vi "海流计数据上传.vi"(8 "错误输入（无错误）":errorcluster) -> (0 "error out":errorcluster)   [LabVIEW 2016, in "数据传输系统-04.lvlib"]
uses:
  <vilib>/Utility/config.llb/Read Key (String).vi
  <vilib>/Utility/config.llb/Write Key (String).vi
  <vilib>/Utility/config.llb/NI_LVConfig.lvlib
  <vilib>/ptbypt/NI_PtbyPt.lvlib
panel:
  out "读取的时间值":string caption="值"
  out "超时":bool
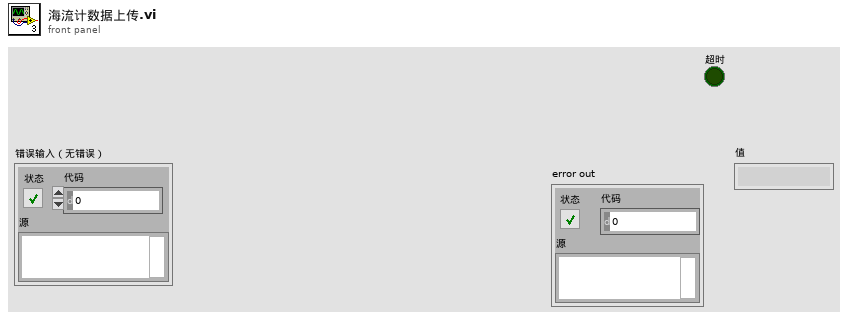
[diagram p1: front panel]
types:
  T1 = enum16{"open", "replace", "create", "open or create", "replace or create", "replace or create with confirmation"}
  T2 = cluster{"setini":string, "sysini":string, "hechaini":string, "actualwrite":string, "actualread":string, "datasent":string, "反控命令信息队列":string, "反控与仪器交互":string}
  T3 = typedef "NI_LVConfig.lvlib/Config Data RefNum.ctl" = refnum<k1>
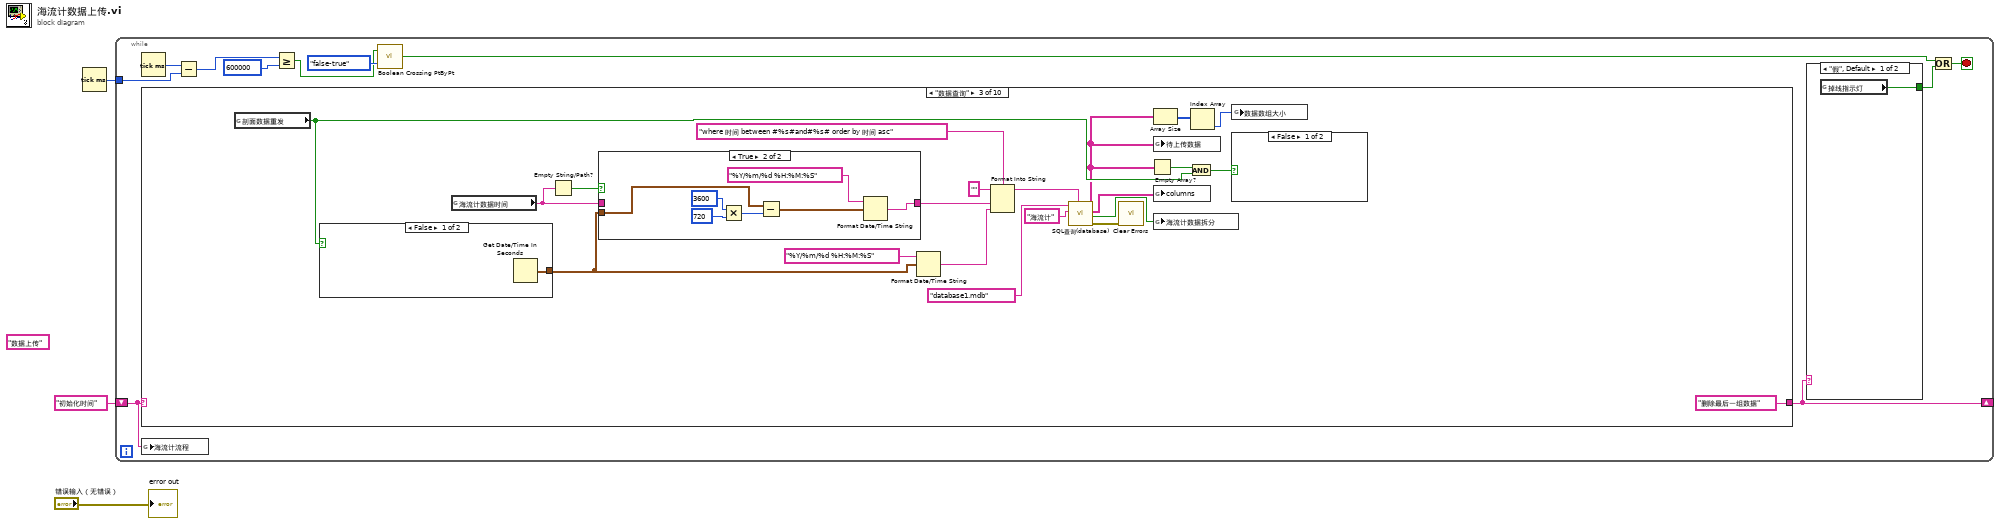
[diagram p0: block diagram]
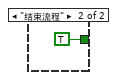
[diagram p2: hidden frame]
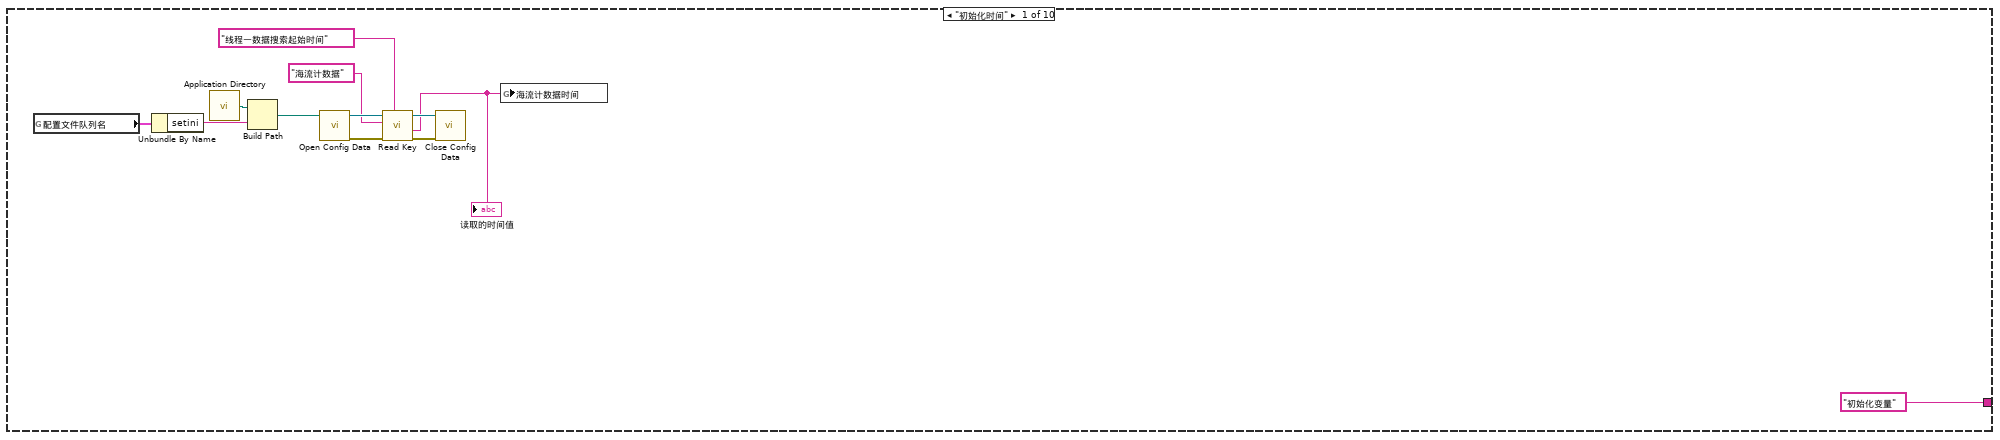
[diagram p3: hidden frame]
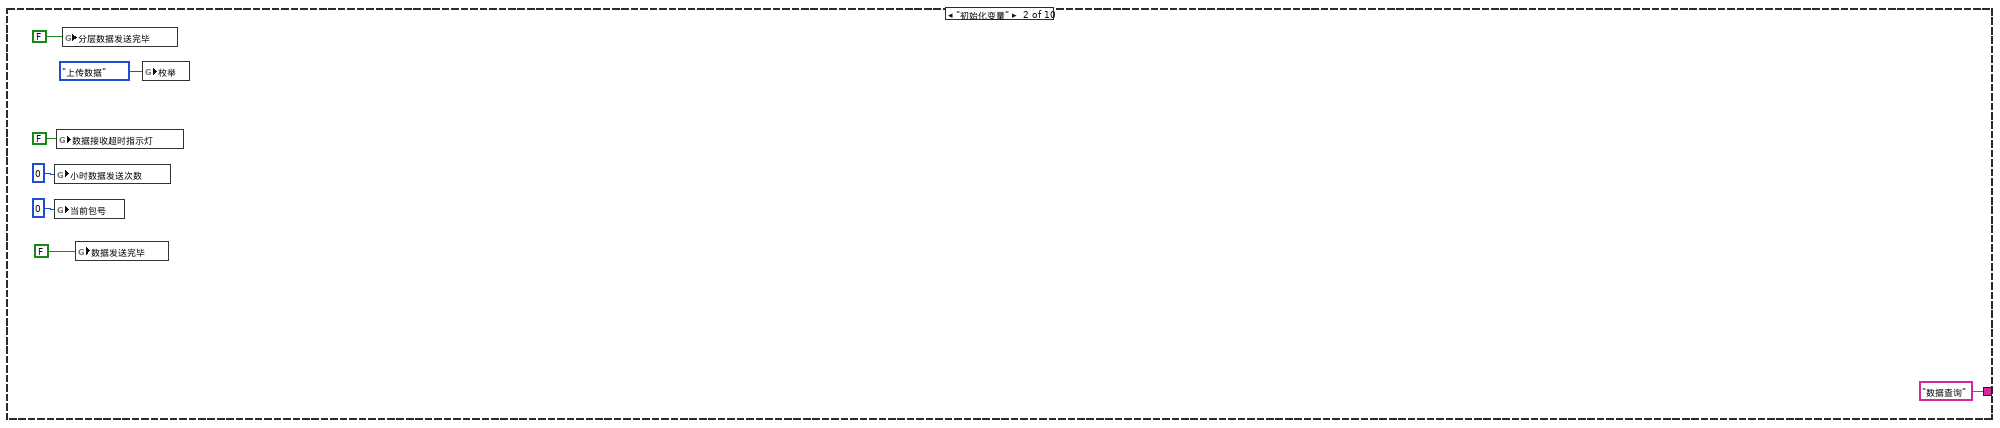
[diagram p4: hidden frame]
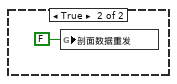
[diagram p5: hidden frame]
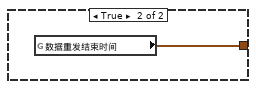
[diagram p7: hidden frame]
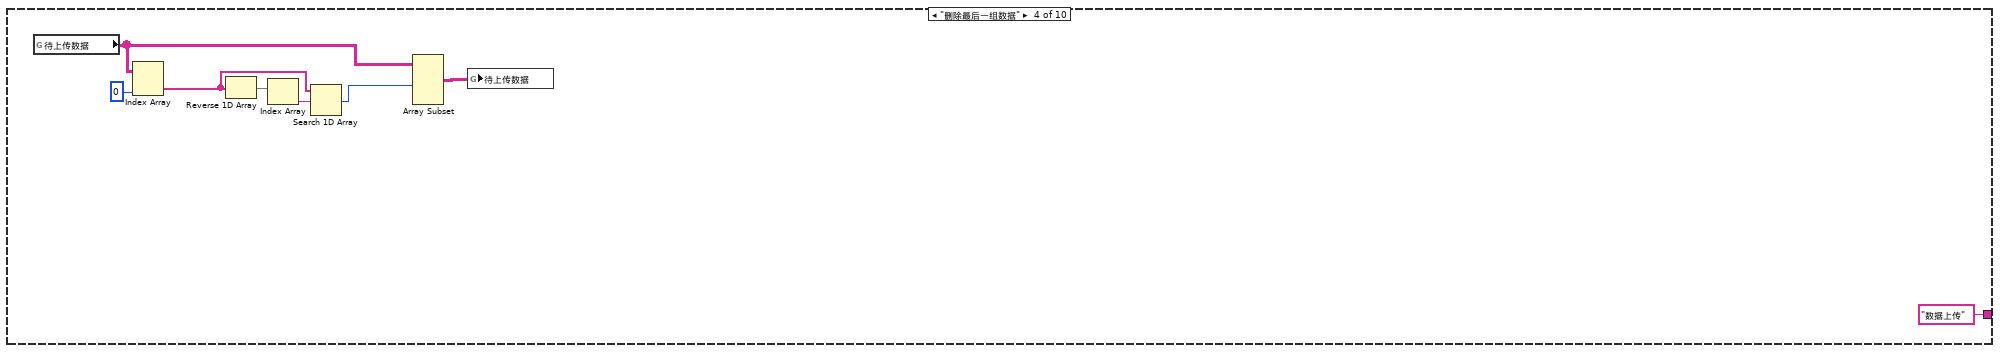
[diagram p8: hidden frame]
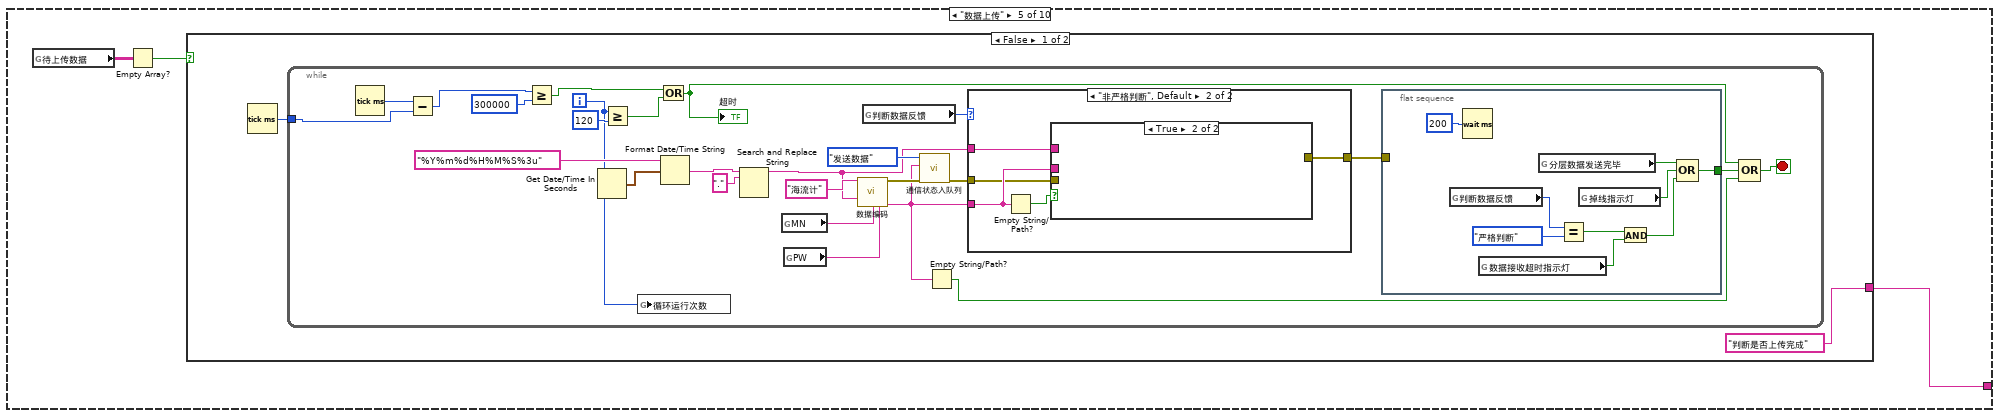
[diagram p9: hidden frame]
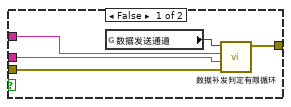
[diagram p11: hidden frame]
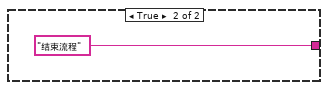
[diagram p12: hidden frame]
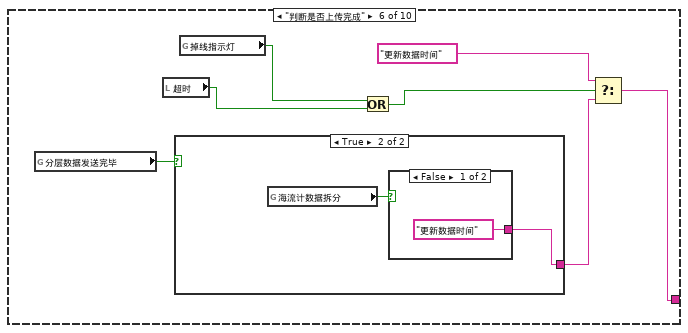
[diagram p13: hidden frame]
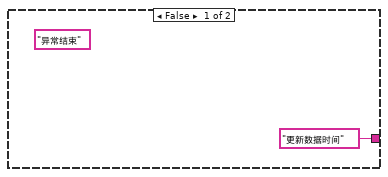
[diagram p14: hidden frame]
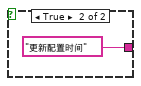
[diagram p15: hidden frame]
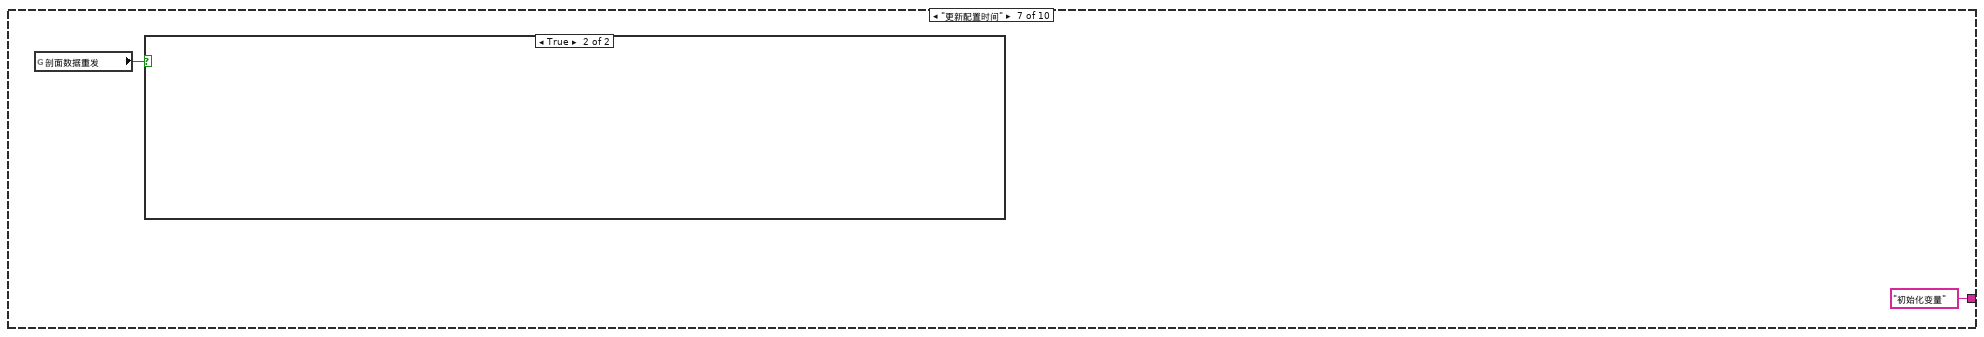
[diagram p16: hidden frame]
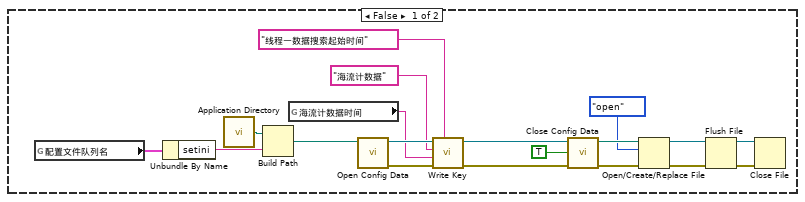
[diagram p17: hidden frame]
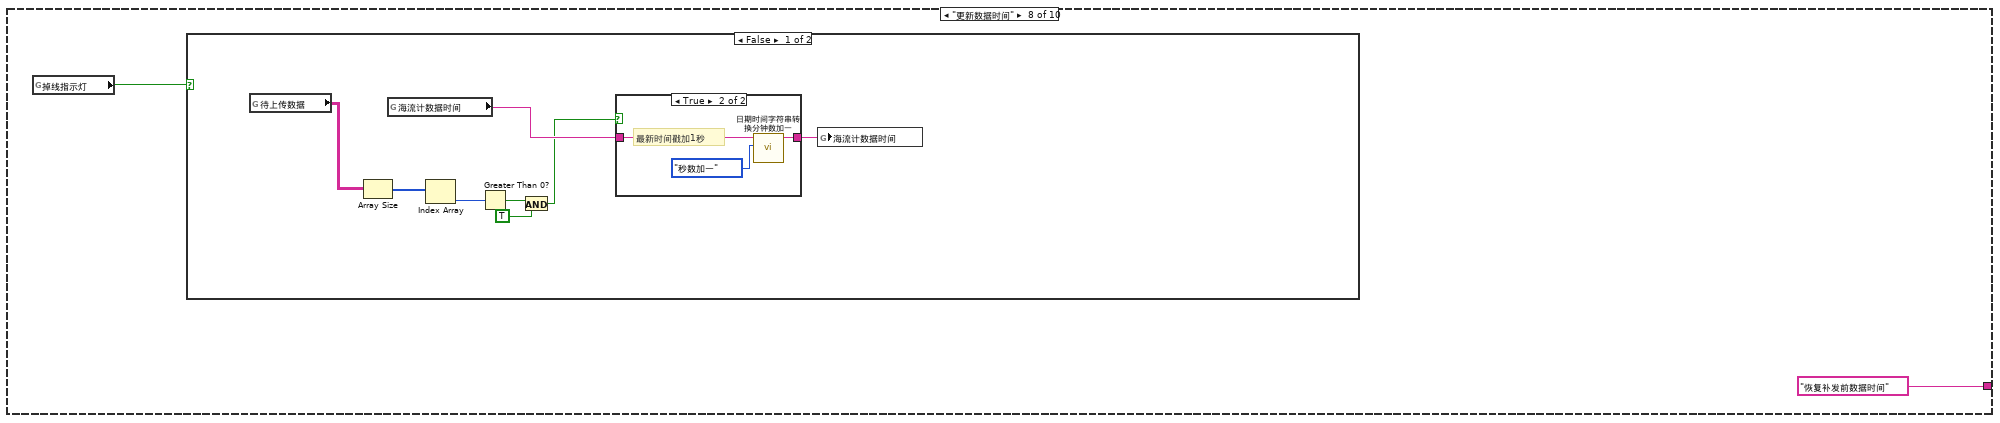
[diagram p18: hidden frame]
diagram:
  (unwired) "数据上传"
  n1 = Tick Count (ms)() -> (millisecond timer value=w2:u32)
  n2 = while {
    shift-right: [w14] -> _
    shift-left: "初始化时间" -> [w13]
    tunnel: w2 -> [w11]
    stop <- w7 stop-if-true
    n3 = Tick Count (ms)() -> (millisecond timer value=w12:u32)
    n4 = case shown="\"数据查询\"" w13 {
      tunnel: ["初始化变量" "数据查询" "删除最后一组数据" "数据上传" w76 w130 "初始化变量" "恢复补发前数据时间" "结束流程" "结束流程"] -> w14
      frame "初始化时间" {
        n5 = global read "全局1.vi" "配置文件队列名"() -> (w28:T2)
        n6 = Unbundle By Name(w28) -> ("setini"=w21:string)
        n7 = call <vilib>:"Application Directory.vi"() -> ("Application Directory"=w22:path)
        n8 = Build Path(base path=w22, name or relative path=w21) -> (appended path=w20:path)
        n9 = call <vilib>:"Open Config Data.vi"("configuration file path"=w20) -> ("error out"=w25:errorcluster, "refnum"=w26:T3)  [unwired: 8 in, 1 out]
        n10 = call-poly <vilib>:"Read Key.vi"("section"="线程一数据搜索起始时间", "error in (no error)"=w25, "key"="海流计数据", "refnum"=w26) -> ("error out"=w23:errorcluster, "value"=w18:string, "refnum out"=w24:T3)  [unwired: 4 in, 1 out]
        "读取的时间值" <- w18
        n11 = call <vilib>:"Close Config Data.vi"("error in (no error)"=w23, "refnum"=w24) -> ()  [unwired: 8 in, 2 out]
        n12 = global write "全局 水样时间.vi" "海流计数据时间"(w18) -> ()
      }
      frame "初始化变量" {
        n13 = global write "全局 小时数据发送次数.vi" "小时数据发送次数"(0 ("小时数据发送次数")) -> ()
        n14 = global write "全局 数据数组大小.vi" "当前包号"(0 ("当前包号")) -> ()
        n15 = global write "全局 数据发送重叠.vi" "数据接收超时指示灯"(FALSE ("数据接收超时指示灯")) -> ()
        n16 = global write "全局 数据数组大小.vi" "分层数据发送完毕"(FALSE ("海流计数据发送完毕")) -> ()
        n17 = global write "全局 数据数组大小.vi" "数据发送完毕"(FALSE ("海流计数据发送完毕")) -> ()
        n18 = global write "全局1.vi" "枚举"(enum16{"返回请求应答", "上传数据", "返回执行结果"}."上传数据" ("枚举")) -> ()
      }
      frame "数据查询" {
        n19 = global read "断电保存全局.vi" "剖面数据重发"() -> (w55:bool)
        n20 = case shown="False" w55 {
          tunnel: [w66 w67] -> w48
          frame False {
            n21 = Get Date/Time In Seconds() -> (seconds since 1Jan1904=w66:timestamp)
          }
          frame True {
            n22 = global read "断电保存全局.vi" "数据重发结束时间"() -> (w67:timestamp)
          }
        }
        n23 = global read "全局 水样时间.vi" "海流计数据时间"() -> (w49:string)
        n24 = Empty String/Path?(string/path=w49) -> (empty?=w47:bool)
        n25 = case shown="True" w47 {
          tunnel: w48 -> [_ w63]
          tunnel: [w58 w59] -> w50
          tunnel: w49 -> [w58 _]
          frame False {
          }
          frame True {
            n26 = Multiply(x=3600, y=720) -> (x*y=w62:i32)
            n27 = Subtract(x=w63, y=w62) -> (x-y=w60:timestamp)
            n28 = Format Date/Time String(time format string (%c)="%Y/%m/%d %H:%M:%S" ("时间格式字符串(%c)"), seconds (now)=w60) -> (date/time string=w59:string)  [unwired: 1 in]
          }
        }
        n29 = Format Date/Time String(time format string (%c)="%Y/%m/%d %H:%M:%S" ("时间格式字符串(%c)"), seconds (now)=w48) -> (date/time string=w41:string)  [unwired: 1 in]
        n30 = Format Into String(format string="where 时间 between #%s#and#%s# order by 时间 asc" ("condition"), initial string="" ("初始字符串"), w50, w41) -> (resulting string=w42:string)  [unwired: 1 in, 1 out]
        n31 = call "SQL查询(database).vi"("condition"=w42, "table输入"="海流计", "database"="database1.mdb") -> ("error out"=w45:errorcluster, "拆分数据"=w52:bool, "columns输出"=w51:string[], "data"=w53:string[][])  [unwired: 5 in]
        n32 = call <vilib>:"Clear Errors.vi"("error in (no error)"=w45) -> ()  [unwired: 5 in, 2 out]
        n33 = Empty Array?(array=w53) -> (empty?=w54:bool)
        n34 = Array Size(array=w53) -> (size(s)=w43:i32[])
        n35 = global write "全局 所有参数.vi" "待上传数据"(w53) -> ()
        n36 = global write "全局 所有参数.vi" "columns"(w51) -> ()
        n37 = global write "全局 所有参数.vi" "海流计数据拆分"(w52) -> ()
        n38 = And(x=w54, y=w55) -> (x .and. y?=w56:bool)
        n39 = Index Array(array=w43) -> (element=w44:i32)  [unwired: 1 in]
        n40 = global write "全局 数据数组大小.vi" "数据数组大小"(w44) -> ()
        n41 = case shown="False" w56 {
          frame False {
          }
          frame True {
            n42 = global write "断电保存全局.vi" "剖面数据重发"(FALSE ("剖面数据重发")) -> ()
          }
        }
      }
      frame "删除最后一组数据" {
        n43 = global read "全局 所有参数.vi" "待上传数据"() -> (w71:string[][])
        n44 = Index Array(array=w71, index (col)=0 ("禁用的索引 (列)")) -> (element=w72:string[])  [unwired: 1 in]
        n45 = Reverse 1D Array(array=w72) -> (reversed array=w74:string[])
        n46 = Index Array(array=w74) -> (element=w73:string)  [unwired: 1 in]
        n47 = Search 1D Array(1D array=w72, element=w73) -> (index of element=w68:i32)  [unwired: 1 in]
        n48 = Array Subset(array=w71, length (row)=w68) -> (w70:string[][])  [unwired: 3 in]
        n49 = global write "全局 所有参数.vi" "待上传数据"(w70) -> ()
      }
      frame "数据上传" {
        n50 = global read "全局 所有参数.vi" "待上传数据"() -> (w77:string[][])
        n51 = Empty Array?(array=w77) -> (empty?=w78:bool)
        n52 = case shown="False" w78 {
          tunnel: ["判断是否上传完成" "结束流程"] -> w76
          frame False {
            n53 = Tick Count (ms)() -> (millisecond timer value=w80:u32)
            n54 = while {
              tunnel: w80 -> [w90]
              i -> [w81]
              stop <- w84 stop-if-true
              n55 = Tick Count (ms)() -> (millisecond timer value=w91:u32)
              n56 = Subtract(x=w91, y=w90) -> (x-y=w92:u32)
              n57 = Greater Or Equal?(x=w92, y=u32 300000) -> (x >= y?=w87:bool)
              n58 = Get Date/Time In Seconds() -> (seconds since 1Jan1904=w104:timestamp)
              n59 = Greater Or Equal?(x=w81, y=120) -> (x >= y?=w86:bool)
              n60 = global write "全局 水样时间.vi" "循环运行次数"(w81) -> ()
              n61 = Or(x=w87, y=w86) -> (x .or. y?=w85:bool)
              "超时" <- w85
              n62 = Format Date/Time String(time format string (%c)="%Y%m%d%H%M%S%3u" ("时间格式字符串(%c)"), seconds (now)=w104) -> (date/time string=w103:string)  [unwired: 1 in]
              n63 = Search and Replace String(input string=w103, search string="." ("搜索字符串")) -> (result string=w96:string)  [unwired: 6 in, 3 out]
              n64 = global read "断电保存全局.vi" "MN"() -> (w98:string)
              n65 = global read "断电保存全局.vi" "PW"() -> (w101:string)
              n66 = call "数据编码.vi"("table输入"="海流计" ("新元素/子数组"), "QN"=w96, "MN"=w98, "PW"=w101) -> ("错误常量"=w100:errorcluster, "通讯包字符串"=w83:string)  [unwired: 10 in]
              n67 = global read "断电保存全局.vi" "判断数据反馈"() -> (w95:enum16{"非严格判断", "严格判断", "不判断"})
              n68 = call "通信状态入队列.vi"("错误输入（无错误）"=w100, "发送报文"=w83, "枚举"=enum16{"打开连接", "发送数据", "读取数据", "数据处理", "关闭连接"}."发送数据") -> ("错误输出"=w97:errorcluster)  [unwired: 8 in]
              n69 = Empty String/Path?(string/path=w83) -> (empty?=w82:bool)
              n70 = case shown="\"非严格判断\", Default" w95 {
                tunnel: [_ w120] -> w94
                tunnel: w83 -> [_ w119]
                tunnel: w96 -> [_ w118]
                tunnel: w97 -> [_ w116]
                frame "不判断" {
                }
                frame "非严格判断", Default {
                  n71 = Empty String/Path?(string/path=w119) -> (empty?=w117:bool)
                  n72 = case shown="True" w117 {
                    tunnel: [w125 _] -> w120
                    tunnel: w119 -> [w124 _]
                    tunnel: w118 -> [w122 _]
                    tunnel: w116 -> [w121 _]
                    frame False {
                      n73 = global read "断电保存全局.vi" "数据发送通道"() -> (w123:enum16{"TCP", "VISA"})
                      n74 = call "数据补发判定有限循环.vi"("错误输入（无错误）"=w121, "数据输入"=w124, "QN"=w122, "数据发送通道"=w123) -> ("error out"=w125:errorcluster)  [unwired: 7 in]
                    }
                    frame True {
                    }
                  }
                }
              }
              n75 = flat-sequence {
                tunnel: w94 -> [_]
                tunnel: [w110] -> w89
                frame #0 {
                  n76 = global read "断电保存全局.vi" "判断数据反馈"() -> (w114:enum16{"非严格判断", "严格判断", "不判断"})
                  n77 = Wait (ms)(milliseconds to wait=u32 200 ("等待时间（毫秒）")) -> ()  [unwired: 1 out]
                  n78 = global read "全局 数据发送重叠.vi" "数据接收超时指示灯"() -> (w107:bool)
                  n79 = global read "全局 数据数组大小.vi" "分层数据发送完毕"() -> (w109:bool)
                  n80 = Equal?(x=w114, y=enum16{"非严格判断", "严格判断", "不判断"}."严格判断") -> (x = y?=w112:bool)
                  n81 = global read "全局 数据发送重叠.vi" "掉线指示灯"() -> (w108:bool)
                  n82 = And(x=w112, y=w107) -> (x .and. y?=w111:bool)
                  n83 = Compound Arithmetic op=OR ("复合运算")(w109, w108, w111) -> (w110:bool)
                }
              }
              n84 = Compound Arithmetic op=OR ("复合运算")(w85, w89, w82) -> (w84:bool)
            }
          }
          frame True {
          }
        }
      }
      frame "判断是否上传完成" {
        n85 = global read "全局 数据数组大小.vi" "分层数据发送完毕"() -> (w133:bool)
        n86 = local read "超时"() -> (w128:bool)
        n87 = case shown="True" w133 {
          tunnel: ["更新数据时间" w135] -> w131
          frame False {
            (unwired) "异常结束"
          }
          frame True {
            n88 = global read "全局 所有参数.vi" "海流计数据拆分"() -> (w136:bool)
            n89 = case shown="False" w136 {
              tunnel: ["更新数据时间" "更新配置时间"] -> w135
              frame False {
              }
              frame True {
              }
            }
          }
        }
        n90 = global read "全局 数据发送重叠.vi" "掉线指示灯"() -> (w129:bool)
        n91 = Or(x=w129, y=w128) -> (x .or. y?=w127:bool)
        n92 = Select(t="更新数据时间", s=w127, f=w131) -> (s? t:f=w130:string)
      }
      frame "更新配置时间" {
        n93 = global read "断电保存全局.vi" "剖面数据重发"() -> (w140:bool)
        n94 = case shown="True" w140 {
          frame False {
            n95 = global read "全局1.vi" "配置文件队列名"() -> (w143:T2)
            n96 = Unbundle By Name(w143) -> ("setini"=w144:string)
            n97 = call <vilib>:"Application Directory.vi"() -> ("Application Directory"=w153:path)
            n98 = Build Path(base path=w153, name or relative path=w144) -> (appended path=w154:path)
            n99 = global read "全局 水样时间.vi" "海流计数据时间"() -> (w145:string)
            n100 = call <vilib>:"Open Config Data.vi"("configuration file path"=w154) -> ("error out"=w156:errorcluster, "refnum"=w155:T3)  [unwired: 8 in, 1 out]
            n101 = call-poly <vilib>:"Write Key.vi"("section"="线程一数据搜索起始时间", "error in (no error)"=w156, "value"=w145, "key"="海流计数据", "refnum"=w155) -> ("error out"=w158:errorcluster, "refnum out"=w157:T3)  [unwired: 4 in, 1 out]
            n102 = call <vilib>:"Close Config Data.vi"("error in (no error)"=w158, "write file if changed (T)"=TRUE, "refnum"=w157) -> ("error out"=w146:errorcluster, "file path"=w147:path)  [unwired: 7 in]
            n103 = Open/Create/Replace File(file path (use dialog)=w147, error in=w146, operation (0:open)=T1."open" ("操作(0:open)")) -> (refnum out=w149:refnum<file>, error out=w148:errorcluster)  [unwired: 3 in, 1 out]
            n104 = Flush File(refnum=w149, error in=w148) -> (refnum out=w150:refnum<file>, error out=w151:errorcluster)
            n105 = Close File(refnum=w150, error in=w151) -> ()  [unwired: 2 out]
          }
          frame True {
          }
        }
      }
      frame "更新数据时间" {
        n106 = global read "全局 数据发送重叠.vi" "掉线指示灯"() -> (w160:bool)
        n107 = case shown="False" w160 {
          frame False {
            n108 = global read "全局 所有参数.vi" "待上传数据"() -> (w163:string[][])
            n109 = Array Size(array=w163) -> (size(s)=w166:i32[])
            n110 = global read "全局 水样时间.vi" "海流计数据时间"() -> (w169:string)
            n111 = Index Array(array=w166) -> (element=w167:i32)  [unwired: 1 in]
            n112 = Greater Than 0?(x=w167) -> (x > 0?=w165:bool)
            n113 = And(x=w165, y=TRUE) -> (x .and. y?=w162:bool)
            n114 = case shown="True" w162 {
              tunnel: [w170 w173] -> w168
              tunnel: w169 -> [w170 w172]
              frame False {
              }
              frame True {
                # "最新时间戳加1秒"
                n115 = call "日期时间字符串转换分钟数加一.vi"("枚举"=enum16{"分钟数加一", "秒数加一", "小时数加一"}."秒数加一", "data[0]"=w172) -> ("日期/时间字符串"=w173:string)  [unwired: 9 in]
              }
            }
            n116 = global write "全局 水样时间.vi" "海流计数据时间"(w168) -> ()
          }
          frame True {
          }
        }
      }
      frame "恢复补发前数据时间" {
        n117 = global read "断电保存全局.vi" "剖面数据重发"() -> (w175:bool)
        n118 = case shown="False" w175 {
          frame False {
            n119 = global read "全局1.vi" "配置文件队列名"() -> (w178:T2)
            n120 = Unbundle By Name(w178) -> ("setini"=w179:string)
            n121 = call <vilib>:"Application Directory.vi"() -> ("Application Directory"=w188:path)
            n122 = Build Path(base path=w188, name or relative path=w179) -> (appended path=w189:path)
            n123 = global read "全局 水样时间.vi" "海流计数据时间"() -> (w180:string)
            n124 = call <vilib>:"Open Config Data.vi"("configuration file path"=w189) -> ("error out"=w191:errorcluster, "refnum"=w190:T3)  [unwired: 8 in, 1 out]
            n125 = call-poly <vilib>:"Write Key.vi"("section"="线程一数据搜索起始时间", "error in (no error)"=w191, "value"=w180, "key"="海流计数据", "refnum"=w190) -> ("error out"=w193:errorcluster, "refnum out"=w192:T3)  [unwired: 4 in, 1 out]
            n126 = call <vilib>:"Close Config Data.vi"("error in (no error)"=w193, "write file if changed (T)"=TRUE, "refnum"=w192) -> ("error out"=w181:errorcluster, "file path"=w182:path)  [unwired: 7 in]
            n127 = Open/Create/Replace File(file path (use dialog)=w182, error in=w181, operation (0:open)=T1."open" ("操作(0:open)")) -> (refnum out=w184:refnum<file>, error out=w183:errorcluster)  [unwired: 3 in, 1 out]
            n128 = Flush File(refnum=w184, error in=w183) -> (refnum out=w185:refnum<file>, error out=w186:errorcluster)
            n129 = Close File(refnum=w185, error in=w186) -> ()  [unwired: 2 out]
          }
          frame True {
            n130 = global write "断电保存全局.vi" "剖面数据重发"(FALSE ("剖面数据重发")) -> ()
            n131 = global read "全局1.vi" "配置文件队列名"() -> (w195:T2)
            n132 = Unbundle By Name(w195) -> ("setini"=w203:string)
            n133 = call <vilib>:"Application Directory.vi"() -> ("Application Directory"=w202:path)
            n134 = Build Path(base path=w202, name or relative path=w203) -> (appended path=w204:path)
            n135 = call <vilib>:"Open Config Data.vi"("configuration file path"=w204) -> ("error out"=w199:errorcluster, "refnum"=w198:T3)  [unwired: 8 in, 1 out]
            n136 = call-poly <vilib>:"Read Key.vi"("section"="线程一数据搜索起始时间", "error in (no error)"=w199, "key"="海流计数据", "refnum"=w198) -> ("error out"=w201:errorcluster, "value"=w206:string, "refnum out"=w200:T3)  [unwired: 4 in, 1 out]
            n137 = call <vilib>:"Close Config Data.vi"("error in (no error)"=w201, "refnum"=w200) -> ()  [unwired: 8 in, 2 out]
            n138 = global write "全局 水样时间.vi" "海流计数据时间"(w206) -> ()
          }
        }
      }
      frame "结束流程", Default {
      }
    }
    n139 = global write "全局 水样时间.vi" "海流计流程"(w13) -> ()
    n140 = Subtract(x=w12, y=w11) -> (x-y=w10:u32)
    n141 = Greater Or Equal?(x=w10, y=u32 600000) -> (x >= y?=w5:bool)
    n142 = call <vilib>:"Boolean Crossing PtByPt.vi"("direction"=enum16{"either", "false-true", "true-false"}."false-true", "input"=w5) -> ("crossing"=w4:bool)  [unwired: 1 in]
    n143 = case shown="\"假\", Default" w14 {
      tunnel: [w15 TRUE] -> w8
      frame "假", Default {
        n144 = global read "全局 数据发送重叠.vi" "掉线指示灯"() -> (w15:bool)
      }
      frame "结束流程" {
      }
    }
    n145 = Or(x=w4, y=w8) -> (x .or. y?=w7:bool)
  }
  "error out" <- "错误输入（无错误）"
